vi "aft_FXLMS SCTL.vi"(4 "control on":bool, 6 "reset? (F)":bool, 7 "filter length":u32=100, 8 "status in":T1, 9 "step size":fxp<+/-,16,-2>=0.009998321533203125, 10 "ref mic":fxp<+/-,24,4>, 11 "error mic":fxp<+/-,24,4>) -> (0 "status out":T1, 3 "y(n)":fxp<+/-,24,4>)   [LabVIEW 2019]
doc: "Contains the settings of a fixed-point LMS adaptive filter.\n\nThis VI is configured as follows:\n\nFilter length: 100\nDefault step size: 9.998322E-3\n\nx(n) word length: 24\nx(n) integer word length: 4\n\nd(n) word length: 24\nd(n) integer word length: 4\n\nw(n) word length: 24\nw(n) integer word length: 4\n\nstep size word length: 16\nstep size integer word length: -2\n\nThe data type of e(n) and y(n) is the same as that of d(n).\n\nTo change the settings of this fixed-point LMS adaptive filter, you must generate LabVIEW FPGA code for this filter again."
uses:
  <vilib>/Platform/TimedLoop/XDataNode/timing_clust.ctl
  <vilib>/Platform/TimedLoop/XDataNode/nitl_modes.ctl
  <vilib>/Platform/TimedLoop/XDataNode/wakeup.ctl
  <vilib>/rvi/DataTransferAndStorage/Container/Common/niFpgaContainerGetUniqueNameForEmu.vi
  <vilib>/rvi/DataTransferAndStorage/Container/Common/niFpgaContainerSetEmuInfo.vi
  <vilib>/rvi/eio/common/nirviEmuReportErrorAndStop.vi
  <vilib>/rvi/Emulation/niFpgaSctlEmulationGetInTimedLoop.vi
  <vilib>/rvi/Emulation/niFpgaEmulationReportErrorSimple.vi
  <vilib>/rvi/Emulation/niFpgaGetClockAttributes.vi
  <vilib>/rvi/Emulation/niFpgaCriticalErrorInLSC.vi
  <vilib>/rvi/Memory/Memory_Emulation/nirvimemoryEmulation.vi
  <vilib>/rvi/Memory/Memory_Emulation/nirvimemoryFastEmulation.vi
  <vilib>/rvi/Memory/Memory_Emulation/niFpgaMemoryEmulationCacheClearOnFirstRun.vi
  <vilib>/rvi/Memory/Memory_Emulation/nirvimemoryEmulationManagerCache_MakeExclusive.vi
  <vilib>/rvi/Memory/Memory_Emulation/niFpgaMemoryEmulationValidateCache.vi
  <vilib>/rvi/Memory/Memory_Emulation/nirvimemoryEmulationManagerCache_InsertValue.vi
  <vilib>/Utility/error.llb/Clear Errors.vi
  <vilib>/rvi/Memory/Memory_Emulation/nirvimemoryEmulationManagerCache_ReleaseExclusive.vi
  <vilib>/rvi/Memory/Memory_Emulation/nirvimemoryEmulationManagerCache_GetValue.vi
  <vilib>/rvi/Emulation/niFpgaEmulationIsFPGAContextNoSignature.vi
  <vilib>/rvi/Memory/Memory_Emulation/nirvimemoryEmulationManagerCache_SetValue.vi
  <vilib>/rvi/Emulation/niFpgaSctlEmulationResourceMgr.vi
  <vilib>/rvi/LocalResourceManager/LocalResourceManager.xnode
  <vilib>/Platform/TimedLoop/XDataNode/XDataNode.xnode
  <vilib>/rvi/DataTransferAndStorage/Container/XNode/niFpgaContainer.xnode
  <vilib>/rvi/FXPMathLib/FxpMul/XNode/nifxpmath_Multiplier.xnode
  <vilib>/rvi/FXPMathLib/FxpSub/XNode/nifxpmath_Sub.xnode
  <vilib>/rvi/FXPMathLib/FxpAdd/XNode/nifxpmath_Add.xnode
  <vilib>/Platform/TimedLoop/XDataNode/XDNodeRunTimeDep.lvlib
  <vilib>/rvi/FXPMathLib/sim/FxpSim.dll
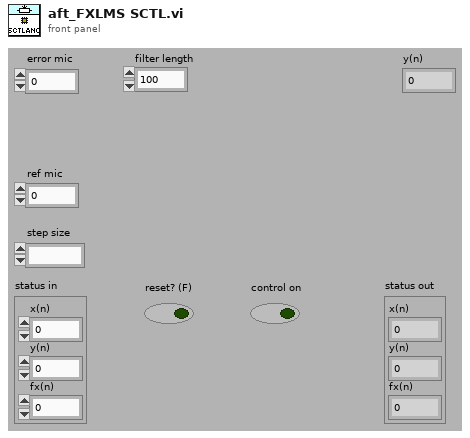
[diagram p1: front panel]
types:
  T1 = cluster{"x(n)":fxp<+/-,32,4>, "fx(n)":fxp<+/-,32,4>, "y(n)":fxp<+/-,32,4>}
  T2 = typedef "XDNodeRunTimeDep.lvlib/timing_clust.ctl" = cluster{"Expected End [f-1]":u64, "Actual End [f-1]":u64, "Finished Late? [f-1]":bool, "Expected End [i-1]":u64, "Actual End [i-1]":u64, "Finished Late? [i-1]":bool, "Expected Start [i]":u64, "Actual Start [i]":u64, "Expected Start [f]":u64, "Actual Start [f]":u64, "Source Name":string, "Structure Name":string, "Period":i64, "Deadline":i64, "Offset":i64, "Start":i64, "Priority":i32, "Timeout":i32, "Mode":T3, "Wakeup Reason":T4, "Error":errorcluster, "Source Type":string, "Secondary Source Type":string, "Global End Time":u64, "Global Start Time":u64, "Frame Duration":u64, "Iteration Duration":u64, "Assigned CPU":i32, "I/O Scan Engine Mode":u32}
  T3 = typedef "XDNodeRunTimeDep.lvlib/nitl_modes.ctl" = enum32{"No Change", "Process missed periods, maintain original phase", "Discard missed periods, maintain original phase", "Process missed periods, ignore original phase", "Discard missed periods, ignore original phase"}
  T4 = typedef "XDNodeRunTimeDep.lvlib/wakeup.ctl" = enum32{"Normal", "Aborted", "Asynchronous wakeup", "Timing source error", "Timed loop error", "Timeout"}
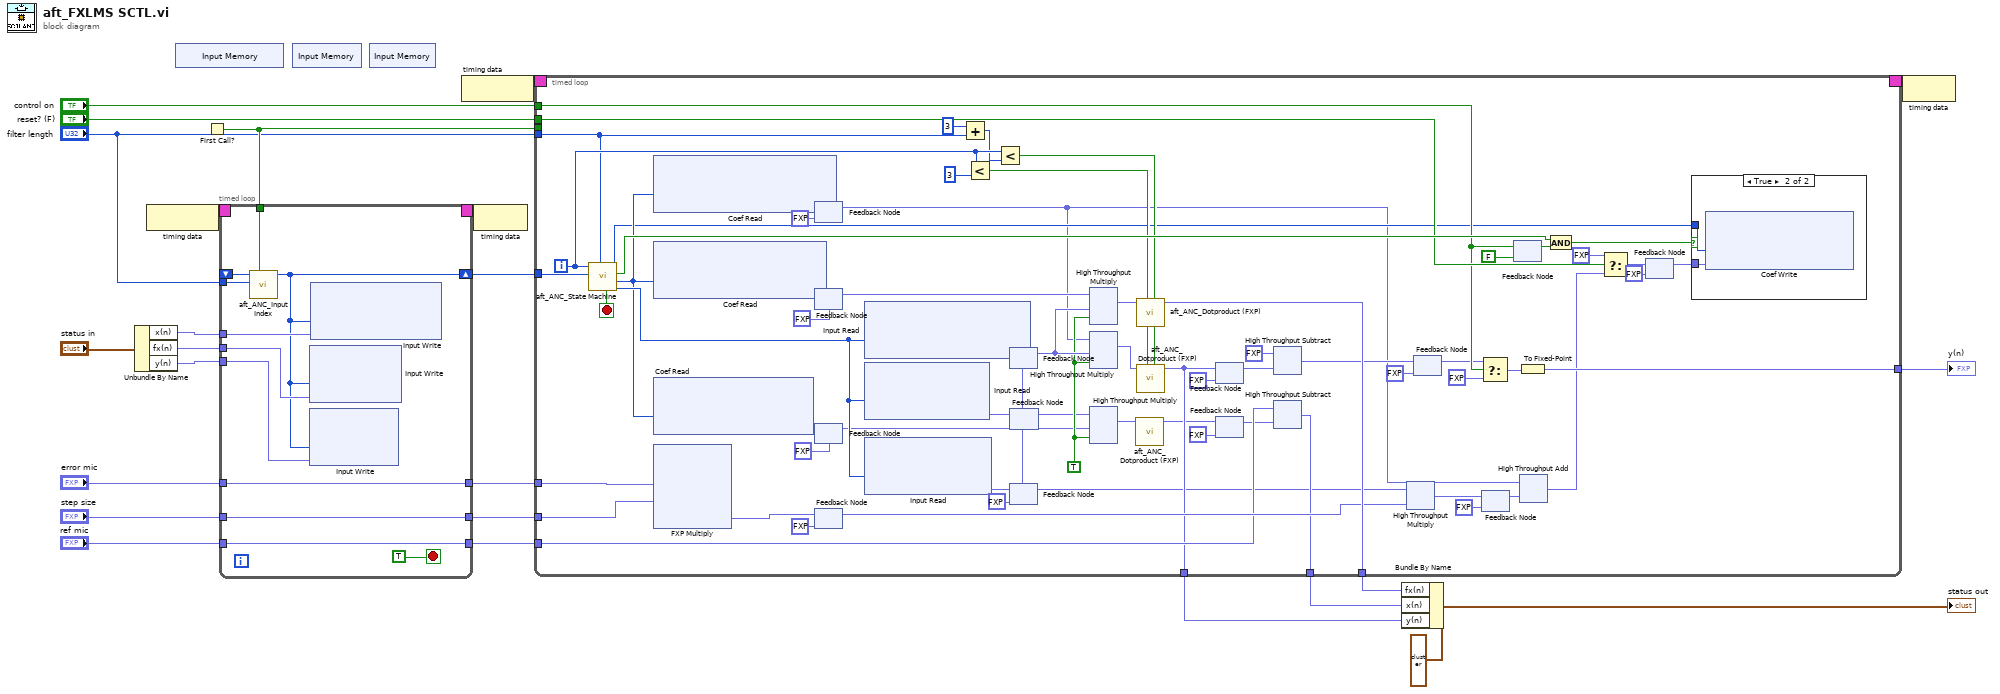
[diagram p0: block diagram]
diagram:
  n1 = Unbundle By Name("status in") -> ("x(n)"=w7:fxp<+/-,32,4>, "fx(n)"=w8:fxp<+/-,32,4>, "y(n)"=w6:fxp<+/-,32,4>)
  n2 = node-c288() -> (w25:T2)
  n3 = xnode ("Input Memory")() -> ()  [unwired: 1 out]
  n4 = First Call?() -> (First Call?: T/F=w17:bool)
  n5 = timed-loop "Pre Loop" {
    timing: w25 -> [_]
    timing-out: [_] -> w24
    tunnel: w17 -> [w35]
    shift-right: [w27] -> w21
    shift-left: _ -> [w34]
    tunnel: "error mic" -> [w33]
    tunnel: [w33] -> w20
    tunnel: "step size" -> [w32]
    tunnel: [w32] -> w18
    tunnel: "ref mic" -> [w30]
    tunnel: "filter length" -> [w31]
    tunnel: [w30] -> w10
    tunnel: w8 -> [w29]
    tunnel: w7 -> [w28]
    tunnel: w6 -> [w26]
    stop <- TRUE stop-if-true
    n6 = call "aft_ANC_Input Index.vi"("first run? (F)"=w35, "filter length"=w31, "state in"=w34) -> ("state out"=w27:u32)  [unwired: 8 out]
    n7 = xnode ("Input Write")("Address"=w27, "Data"=w29) -> ()  [unwired: 1 in, 1 out]
    n8 = xnode ("Input Write")("Address"=w27, "Data"=w26) -> ()  [unwired: 1 in, 1 out]
    n9 = xnode ("Input Write")("Address"=w27, "Data"=w28) -> ()  [unwired: 1 in, 1 out]
  }
  n10 = xnode ("Input Memory")() -> ()  [unwired: 1 out]
  n11 = xnode ("Input Memory")() -> ()  [unwired: 1 out]
  n12 = node-c288() -> (w23:T2)
  n13 = node-c288(w24) -> ()
  n14 = timed-loop "Main Loop" {
    timing: w23 -> [_]
    timing-out: [_] -> w22
    tunnel: w21 -> [w103]
    tunnel: w20 -> [w86]
    tunnel: w18 -> [w92]
    tunnel: w17 -> [_]
    tunnel: "reset? (F)" -> [w102]
    tunnel: "control on" -> [w97]
    tunnel: [w88] -> w14
    tunnel: [w96] -> w2
    tunnel: "filter length" -> [w87]
    tunnel: w10 -> [w83]
    tunnel: [w82] -> w1
    tunnel: [w81] -> w3
    i -> [w101]
    stop <- w99 stop-if-true
    w55 = TRUE ("input valid")
    w56 = fxp<+/-,32,4> 0.0 ("Data")
    n15 = call "aft_ANC_State Machine.vi"("filter length"=w87, "initialize x read address"=w103, "index"=w101) -> ("x read address"=w104:u32, "coefficient read address"=w85:u32, "coefficient write enable"=w105:bool, "coefficient write address"=w47:u32, "stop"=w99:bool)  [unwired: 1 in, 3 out]
    n16 = xnode ("Coef Read")("Address"=w85) -> ("Data"=w98:fxp<+/-,32,4>)  [unwired: 1 in, 1 out]
    n17 = xnode ("Coef Read")("Address"=w85) -> ("Data"=w90:fxp<+/-,32,4>)  [unwired: 1 in, 1 out]
    n18 = xnode ("Coef Read")("Address"=w85) -> ("Data"=w84:fxp<+/-,32,4>)  [unwired: 1 in, 1 out]
    n19 = xnode "FXP Multiply"("x"=w86, "y"=w92) -> ("x*y"=w91:fxp<+/-,32,2>)
    n20 = feedback-in #1(w98) -> ()
    n21 = feedback #1(fxp<+/-,32,4> 0.0 ("Data")) -> (w43:fxp<+/-,32,4>)
    n22 = feedback-in #2(w90) -> ()
    n23 = feedback #2(fxp<+/-,32,4> 0.0 ("Data")) -> (w100:fxp<+/-,32,4>)
    n24 = feedback-in #3(w84) -> ()
    n25 = feedback #3(fxp<+/-,32,4> 0.0 ("Data")) -> (w44:fxp<+/-,32,4>)
    n26 = feedback-in #4(w91) -> ()
    n27 = feedback #4(fxp<+/-,32,2> 0.0 ("data out")) -> (w94:fxp<+/-,32,2>)
    n28 = xnode ("Input Read")("Address"=w104) -> ("Data"=w80:fxp<+/-,32,4>)  [unwired: 1 in, 1 out]
    n29 = xnode ("Input Read")("Address"=w104) -> ("Data"=w57:fxp<+/-,32,4>)  [unwired: 1 in, 1 out]
    n30 = xnode ("Input Read")("Address"=w104) -> ("Data"=w58:fxp<+/-,32,4>)  [unwired: 1 in, 1 out]
    n31 = Add(x=u32 3, y=w87) -> (x+y=w77:u32)
    n32 = Less?(x=w101, y=3) -> (x < y?=w76:bool)
    n33 = Less?(x=w101, y=w77) -> (x < y?=w75:bool)
    n34 = feedback-in #5(w80) -> ()
    n35 = feedback #5(w56) -> (w66:fxp<+/-,32,4>)
    n36 = feedback-in #6(w58) -> ()
    n37 = feedback #6(w56) -> (w72:fxp<+/-,32,4>)
    n38 = feedback-in #7(w57) -> ()
    n39 = feedback #7(w56) -> (w45:fxp<+/-,32,4>)
    n40 = xnode "High Throughput Multiply"("x"=w100, "y"=w66, "input valid"=w55) -> ("x*y"=w62:fxp<+/-,64,4>)  [unwired: 1 in, 2 out]
    n41 = xnode "High Throughput Multiply"("x"=w43, "y"=w66, "input valid"=w55) -> ("x*y"=w61:fxp<+/-,64,4>)  [unwired: 1 in, 2 out]
    n42 = xnode "High Throughput Multiply"("x"=w45, "y"=w44, "input valid"=w55) -> ("x*y"=w54:fxp<+/-,64,4>)  [unwired: 1 in, 2 out]
    n43 = call "aft_ANC_Dotproduct (FXP).vi"("data in"=w54) -> ("data out"=w52:fxp<+/-,32,4>)  [unwired: 4 in, 6 out]
    n44 = call "aft_ANC_Dotproduct (FXP).vi"("enable(F)"=w75, "reset(F)"=w76, "data in"=w62) -> ("data out"=w96:fxp<+/-,32,4>)  [unwired: 2 in, 6 out]
    n45 = call "aft_ANC_Dotproduct (FXP).vi"("enable(F)"=w75, "reset(F)"=w76, "data in"=w61) -> ("data out"=w81:fxp<+/-,32,4>)  [unwired: 2 in, 6 out]
    n46 = feedback-in #8(w81) -> ()
    n47 = feedback #8(fxp<+/-,32,4> 0.0 ("Data")) -> (w59:fxp<+/-,32,4>)
    n48 = feedback-in #9(w52) -> ()
    n49 = feedback #9(fxp<+/-,32,4> 0.0 ("Data")) -> (w51:fxp<+/-,32,4>)
    n50 = xnode "High Throughput Subtract"("x"=fxp<+/-,32,4> 0.0 ("Data"), "y"=w59) -> ("x-y"=w65:fxp<+/-,32,4>)
    n51 = xnode "High Throughput Subtract"("x"=w83, "y"=w51) -> ("x-y"=w82:fxp<+/-,32,4>)
    n52 = xnode "High Throughput Multiply"("x"=w72, "y"=w94) -> ("x*y"=w71:fxp<+/-,32,2>)
    n53 = feedback-in #10(w65) -> ()
    n54 = feedback #10(fxp<+/-,32,4> 0.0 ("Data")) -> (w64:fxp<+/-,32,4>)
    n55 = Select(t=w64, s=w97, f=fxp<+/-,32,4> 0.0 ("Data")) -> (s? t:f=w89:fxp<+/-,32,4>)
    n56 = feedback-in #11(w71) -> ()
    n57 = feedback #11(fxp<+/-,32,2> 0.0) -> (w42:fxp<+/-,32,2>)
    n58 = feedback-in #12(w97) -> ()
    n59 = feedback #12(FALSE ("control on")) -> (w49:bool)
    n60 = To Fixed-Point(number=w89) -> (fixed-point=w88:fxp<+/-,24,4>)  [unwired: 1 out]
    n61 = xnode "High Throughput Add"("x"=w43, "y"=w42) -> ("x+y"=w70:fxp<+/-,32,4>)
    n62 = And(x=w105, y=w49) -> (x .and. y?=w48:bool)
    n63 = Select(t=fxp<+/-,32,4> 0.0 ("Data"), s=w102, f=w70) -> (s? t:f=w69:fxp<+/-,32,4>)
    n64 = feedback-in #13(w69) -> ()
    n65 = feedback #13(fxp<+/-,32,4> 0.0 ("Data")) -> (w67:fxp<+/-,32,4>)
    n66 = case "coef write case" shown="True" w48 {
      tunnel: w47 -> [_ w107]
      tunnel: w67 -> [_ w106]
      frame False {
      }
      frame True {
        n67 = xnode ("Coef Write")("Address"=w107, "Data"=w106) -> ()  [unwired: 1 in, 1 out]
      }
    }
  }
  "y(n)" <- w14
  n68 = Bundle By Name(cluster=T1 {"x(n)"=0.0, "fx(n)"=0.0, "y(n)"=0.0} ("status out 2"), "fx(n)"=w2, "x(n)"=w1, "y(n)"=w3) -> (→"status out":T1)
  n69 = node-c288(w22) -> ()
